vi "LUCS001RT_GPS_RS232_GetU16_Data.vi"(1 "N-Bytes":u8[](array[numeric])=[96, 57, 252, 15, 42, 208, 229, 185, 4, 137, 9, 20, 84, 3, 3, 0, 255, 136, 3, 0, 136, 15, 0, 0, 223, 21, 0, 0, 116, 9] format="%02x", 3 "index":i32) -> (0 "U16":u16)   [LabVIEW 2024]
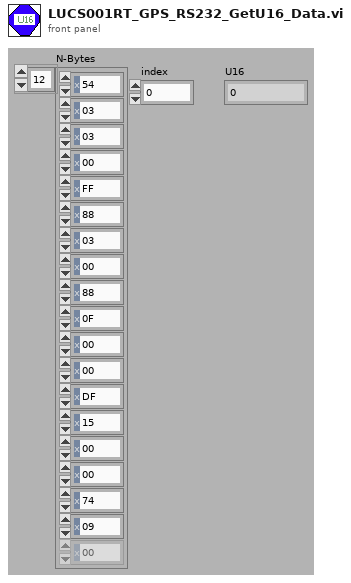
[diagram p1: front panel]
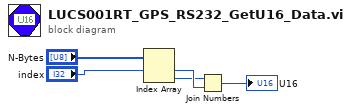
[diagram p0: block diagram]
diagram:
  n1 = Index Array(array="N-Bytes", index #1="index") -> (element #1=w3:u8, element #2=w2:u8)  [unwired: 1 in]
  n2 = Join Numbers(hi=w2, lo=w3) -> ((hi.lo)=→"U16":u16)
